vi "Set Ready to Send.vi"(8 "error in (no error)":errorcluster, 11 "TCP_Streamer in":refnum<class "TCP_Streamer_Publisher.lvclass">) -> (0 "error out":errorcluster, 3 "TCP_Streamer out":refnum<class "TCP_Streamer_Publisher.lvclass">)   [LabVIEW 2021, in "TCP_Streamer_Publisher.lvclass"]
doc: "Set that data is ready to send. \nNormally the state is a read-only parameter. This allows setting the state that data is now ready to send in the state machine."
uses:
  TCP_Streamer_Publisher.lvclass
  Typedef/State.ctl
  TCP_Streamer_Publisher.lvclass/TCP_Streamer_Publisher.ctl
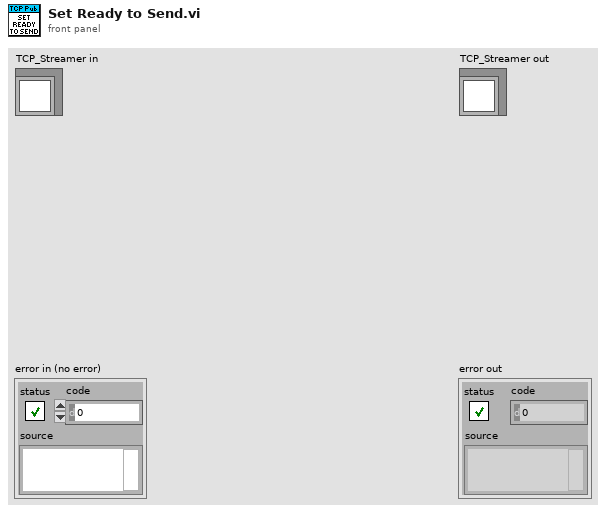
[diagram p1: front panel]
types:
  T1 = typedef "TCP_Streamer_Publisher.lvclass/State.ctl" = enum16{"Stopped", "Listening", "Ready for Data", "Ready to Send", "Sending"}
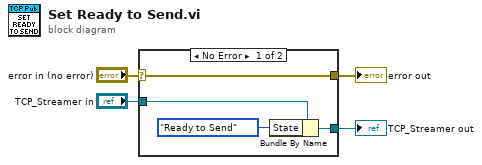
[diagram p0: block diagram]
diagram:
  n1 = case shown="No Error" "error in (no error)" {
    selector: "error in (no error)" -> [w8 w10]
    tunnel: [w8 w10] -> w3
    tunnel: [w5 w9] -> w1
    tunnel: "TCP_Streamer in" -> [w7 w9]
    frame No Error {
      n2 = Bundle By Name(cluster=w7, "State"=State."Ready to Send") -> (w5:refnum<class "TCP_Streamer_Publisher.lvclass">)
    }
    frame Error {
    }
  }
  "error out" <- w3
  "TCP_Streamer out" <- w1
